vi "Get Image.vi"(8 "error in (no error)":errorcluster, 10 "Cluster":T2 {"Camera Settings"."VideoMode" items=["640 x 480 YUY 2 30.00 fps", "640 x 480 YUY 2 20.00 fps", "640 x 480 YUY 2 15.00 fps", "640 x 480 YUY 2 10.00 fps", "640 x 480 YUY 2 7.50 fps", "1280 x 720 YUY 2 10.00 fps", "1280 x 720 YUY 2 7.50 fps", "960 x 544 YUY 2 15.00 fps", "960 x 544 YUY 2 10.00 fps", "960 x 544 YUY 2 7.50 fps", "800 x 448 YUY 2 20.00 fps", "800 x 448 YUY 2 15.00 fps", "800 x 448 YUY 2 10.00 fps", "800 x 448 YUY 2 7.50 fps", "640 x 360 YUY 2 30.00 fps", "640 x 360 YUY 2 20.00 fps", "640 x 360 YUY 2 15.00 fps", "640 x 360 YUY 2 10.00 fps", "640 x 360 YUY 2 7.50 fps", "424 x 240 YUY 2 30.00 fps", "424 x 240 YUY 2 20.00 fps", "424 x 240 YUY 2 15.00 fps", "424 x 240 YUY 2 10.00 fps", "424 x 240 YUY 2 7.50 fps", "352 x 288 YUY 2 30.00 fps", "352 x 288 YUY 2 20.00 fps", "352 x 288 YUY 2 15.00 fps", "352 x 288 YUY 2 10.00 fps", "352 x 288 YUY 2 7.50 fps", "320 x 240 YUY 2 30.00 fps", "320 x 240 YUY 2 20.00 fps", "320 x 240 YUY 2 15.00 fps", "320 x 240 YUY 2 10.00 fps", "320 x 240 YUY 2 7.50 fps", "800 x 600 YUY 2 15.00 fps", "800 x 600 YUY 2 10.00 fps", "800 x 600 YUY 2 7.50 fps", "176 x 144 YUY 2 30.00 fps", "176 x 144 YUY 2 20.00 fps", "176 x 144 YUY 2 15.00 fps", "176 x 144 YUY 2 10.00 fps", "176 x 144 YUY 2 7.50 fps", "160 x 120 YUY 2 30.00 fps", "160 x 120 YUY 2 20.00 fps", "160 x 120 YUY 2 15.00 fps", "160 x 120 YUY 2 10.00 fps", "160 x 120 YUY 2 7.50 fps", "1280 x 800 YUY 2 10.00 fps", "640 x 480 JPEG 30.00 fps", "640 x 480 JPEG 20.00 fps", "640 x 480 JPEG 15.00 fps", "640 x 480 JPEG 10.00 fps", "640 x 480 JPEG 7.50 fps", "1280 x 720 JPEG 30.00 fps", "1280 x 720 JPEG 20.00 fps", "1280 x 720 JPEG 15.00 fps", "1280 x 720 JPEG 10.00 fps", "1280 x 720 JPEG 7.50 fps", "960 x 544 JPEG 30.00 fps", "960 x 544 JPEG 20.00 fps", "960 x 544 JPEG 15.00 fps", "960 x 544 JPEG 10.00 fps", "960 x 544 JPEG 7.50 fps", "800 x 448 JPEG 30.00 fps", "800 x 448 JPEG 20.00 fps", "800 x 448 JPEG 15.00 fps", "800 x 448 JPEG 10.00 fps", "800 x 448 JPEG 7.50 fps", "640 x 360 JPEG 30.00 fps", "640 x 360 JPEG 20.00 fps", "640 x 360 JPEG 15.00 fps", "640 x 360 JPEG 10.00 fps", "640 x 360 JPEG 7.50 fps", "800 x 600 JPEG 30.00 fps", "800 x 600 JPEG 20.00 fps", "800 x 600 JPEG 15.00 fps", "800 x 600 JPEG 10.00 fps", "800 x 600 JPEG 7.50 fps", "416 x 240 JPEG 30.00 fps", "416 x 240 JPEG 20.00 fps", "416 x 240 JPEG 15.00 fps", "416 x 240 JPEG 10.00 fps", "416 x 240 JPEG 7.50 fps", "352 x 288 JPEG 30.00 fps", "352 x 288 JPEG 20.00 fps", "352 x 288 JPEG 15.00 fps", "352 x 288 JPEG 10.00 fps", "352 x 288 JPEG 7.50 fps", "176 x 144 JPEG 30.00 fps", "176 x 144 JPEG 20.00 fps", "176 x 144 JPEG 15.00 fps", "176 x 144 JPEG 10.00 fps", "176 x 144 JPEG 7.50 fps", "320 x 240 JPEG 30.00 fps", "320 x 240 JPEG 20.00 fps", "320 x 240 JPEG 15.00 fps", "320 x 240 JPEG 10.00 fps", "320 x 240 JPEG 7.50 fps", "160 x 120 JPEG 30.00 fps", "160 x 120 JPEG 20.00 fps", "160 x 120 JPEG 15.00 fps", "160 x 120 JPEG 10.00 fps", "160 x 120 JPEG 7.50 fps"]}, 11 "Refnum in":T1) -> (0 "error out":errorcluster, 3 "Refnum out":T1)   [LabVIEW 2015]
uses:
  Camera Data.ctl
  <vilib>/userdefined/High Color/IMAQdx.ctl
  Camera Settings.ctl
  Support Vision Code/38 Video Mode.ctl
  <vilib>/vision/Image Controls.llb/IMAQ Image.ctl
  <vilib>/vision/driver/NI_Vision_Acquisition_Software.lvlib
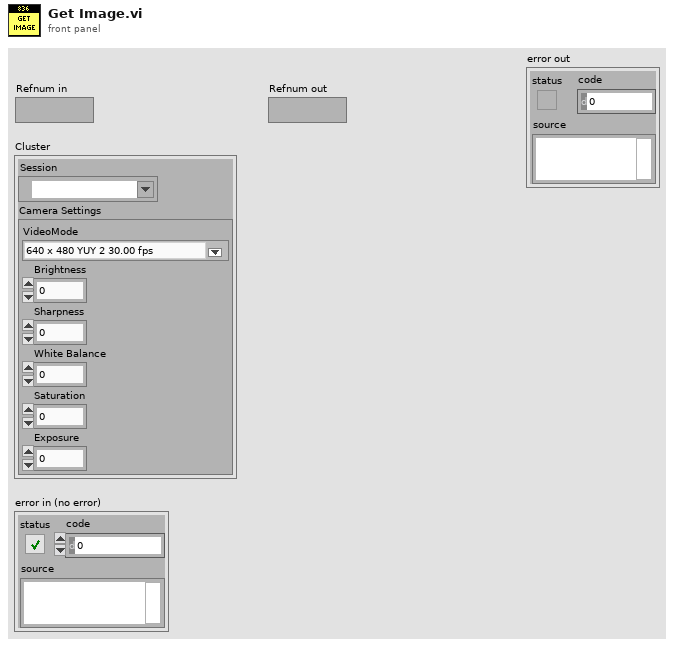
[diagram p1: front panel]
types:
  T1 = typedef "IMAQ Image.ctl" = refnum<image>
  T2 = typedef "Camera Data.ctl" = cluster{"Session":T3, "Camera Settings":T4}
  T3 = typedef "IMAQdx.ctl" = refnum<k21>
  T4 = typedef "Camera Settings.ctl" = cluster{"VideoMode":T5, "Brightness":i32, "Sharpness":i32, "White Balance":i32, "Saturation":i32, "Exposure":i32}
  T5 = typedef "38 Video Mode.ctl" = u32
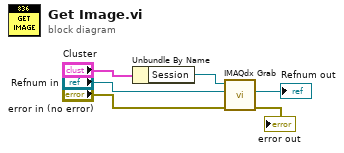
[diagram p0: block diagram]
diagram:
  n1 = Unbundle By Name("Cluster") -> ("Session"=w6:T3)
  n2 = call <vilib>:"IMAQdx Grab.vi"("error in"="error in (no error)", "Image In"="Refnum in", "Session In"=w6) -> ("error out"=→"error out":errorcluster, "Image Out"=→"Refnum out":T1)  [unwired: 5 in, 2 out]
